vi "GFBuildMagTriggerWaveFormSLiC.vi"(1 "Li Trig Time":dbl, 2 "Li On Width":dbl, 4 "LED Trig Time":dbl, 6 "Invert":bool, 7 "LED On Width":dbl, 8 "error in":errorcluster, 9 "Enable Array":bool[](array[boolean])=[TRUE, TRUE, TRUE, TRUE, TRUE, TRUE, TRUE], 10 "Chan Delays":dbl[](array[numeric])=[-0.8, -0.9, -0.7] format="%.6f", 11 "task in":refnum<k21>="USB-MagAndTrigFire") -> (0 "error out":errorcluster, 3 "task out":refnum<k21>="USB-MagAndTrigFire", 5 "Digital Waveform Graph":digitalwaveform[](graph))   [LabVIEW 2016]
doc: "Magnet timing pulses should be input relative to fast fire pulse, at most 2 s behind (-2 to 0 s)"
uses:
  <vilib>/Waveform/DWDTOps.llb/DWDT Boolean Array to Digital.vi
  <resource>/objmgr/daqmx.rc
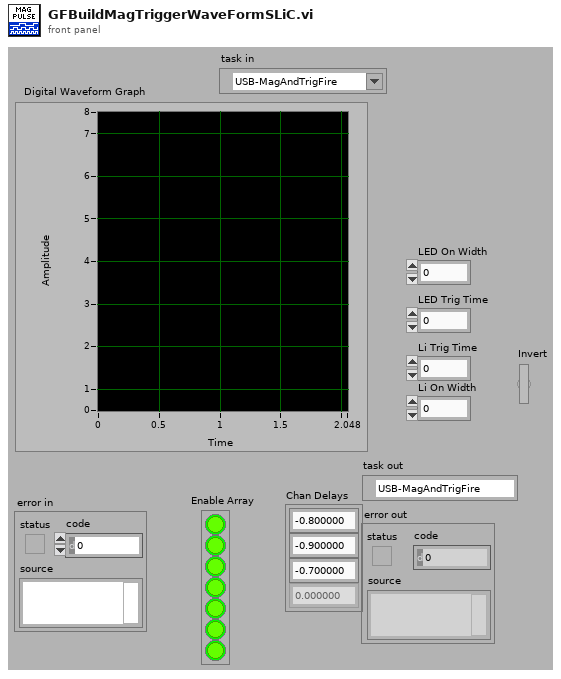
[diagram p1: front panel]
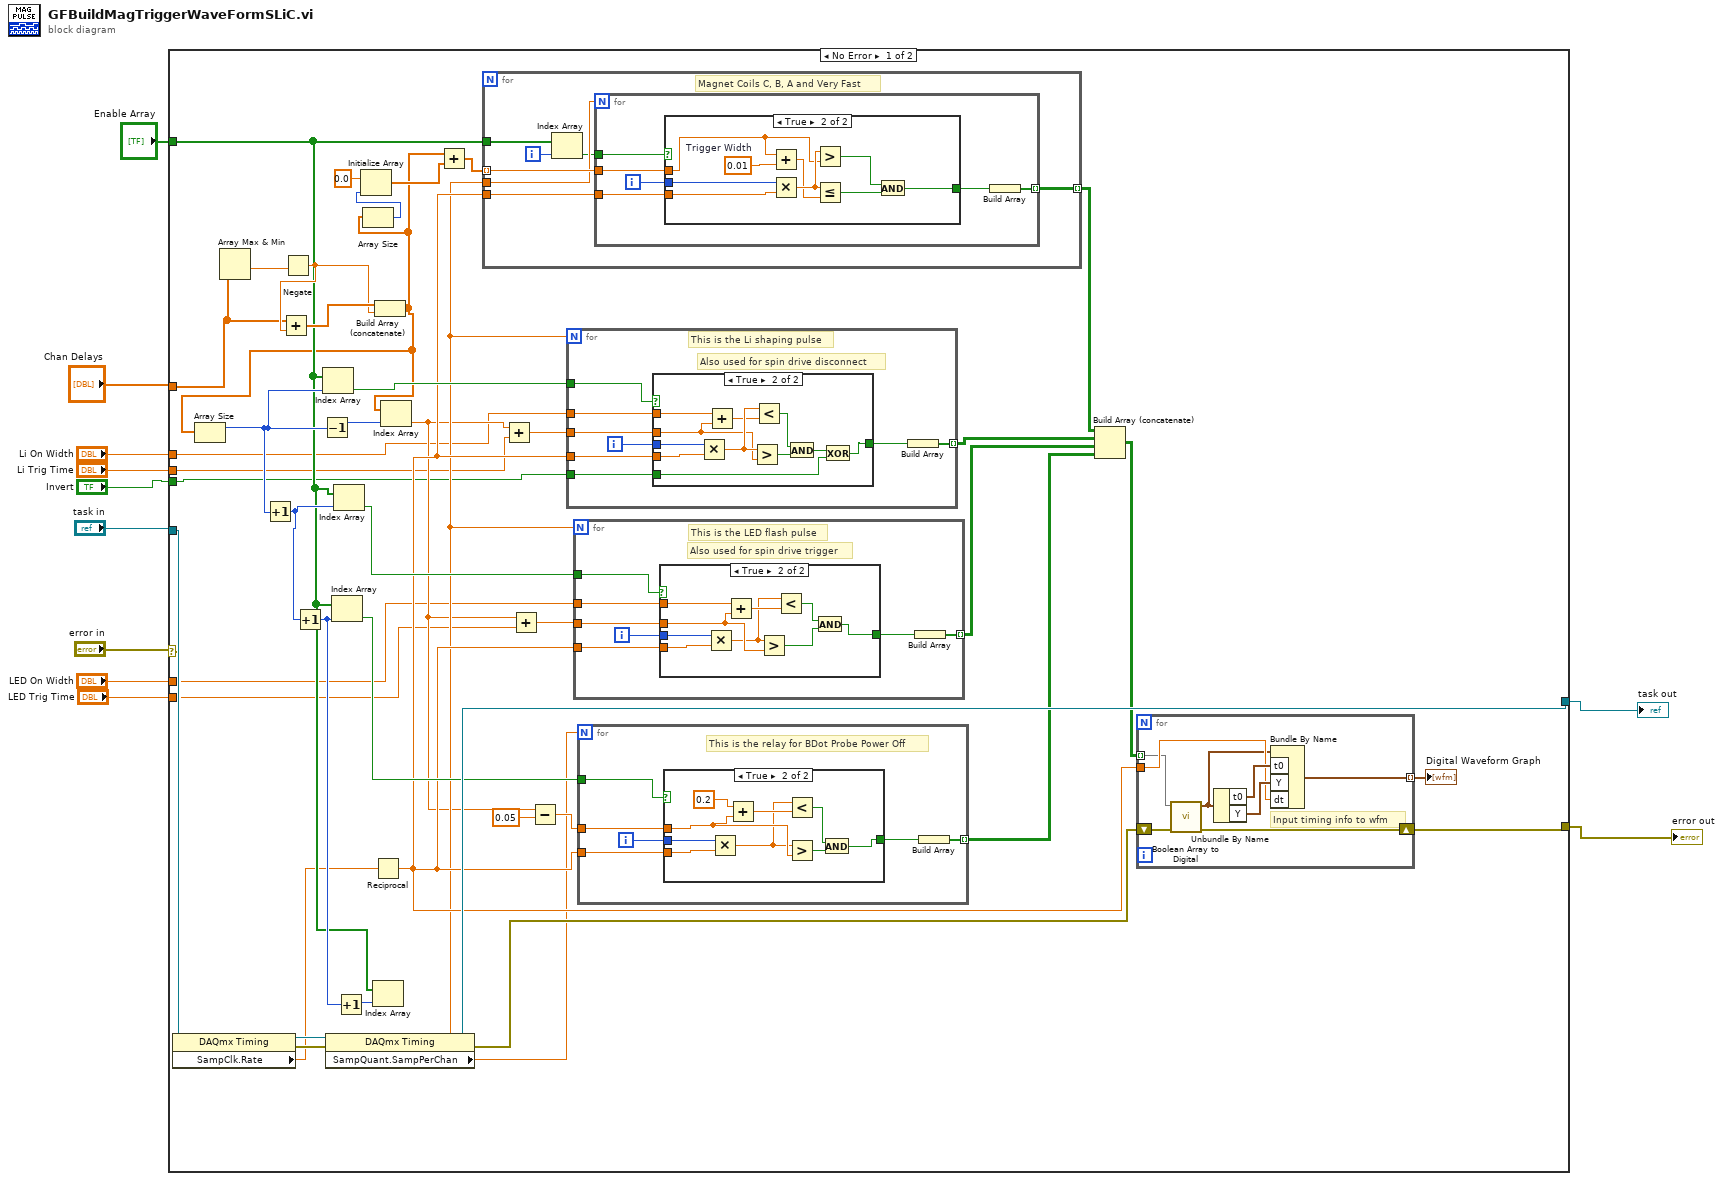
[diagram p0: block diagram]
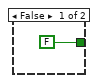
[diagram p2: hidden frame]
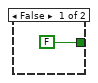
[diagram p3: hidden frame]
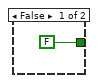
[diagram p4: hidden frame]
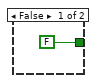
[diagram p5: hidden frame]
diagram:
  n1 = case shown="No Error" "error in" {
    selector: "error in" -> [w52 w140]
    tunnel: "task in" -> [w53 w141]
    tunnel: [w49 w141] -> w10
    tunnel: [w55 w140] -> w8
    tunnel: "Chan Delays" -> [w19 _]
    tunnel: "Enable Array" -> [w26 _]
    tunnel: "LED Trig Time" -> [w17 _]
    tunnel: "LED On Width" -> [w15 _]
    tunnel: "Li Trig Time" -> [w14 _]
    tunnel: "Li On Width" -> [w13 _]
    tunnel: "Invert" -> [w12 _]
    frame No Error {
      n2 = property class="DAQmx Timing"(reference=w53, error in=w52) -> (reference out=w51:refnum<k21>, error out=w50:errorcluster, "SampClk.Rate"=w25:dbl)
      n3 = Array Max & Min(array=w19) -> (min value=w45:dbl)  [unwired: 3 out]
      n4 = Negate(x=w45) -> (-x=w43:dbl)
      n5 = Add(x=w19, y=w43) -> (x+y=w44:dbl[])
      n6 = property class="DAQmx Timing"(reference=w51, error in=w50) -> (reference out=w49:refnum<k21>, error out=w37:errorcluster, "SampQuant.SampPerChan"=w29:dbl)
      n7 = Reciprocal(x=w25) -> (1/x=w33:dbl)
      n8 = Build Array (concatenate)(w44, w43) -> (w22:dbl[])
      n9 = Array Size(array=w22) -> (size(s)=w32:i32)
      n10 = Increment(x=w32) -> (x+1=w38:i32)
      n11 = Increment(x=w38) -> (x+1=w27:i32)
      n12 = Decrement(x=w32) -> (x-1=w48:i32)
      n13 = Index Array(array=w26, index=w32) -> (element=w42:bool)
      n14 = Index Array(array=w26, index=w27) -> (element=w36:bool)
      n15 = Index Array(array=w26, index=w38) -> (element=w40:bool)
      n16 = Increment(x=w27) -> (x+1=w28:i32)
      n17 = Array Size(array=w22) -> (size(s)=w21:i32)
      n18 = Initialize Array(0.0 ("element"), w21) -> (w23:dbl[])
      n19 = Index Array(array=w26, index=w28) -> ()  [unwired: 1 out]
      n20 = Index Array(array=w22, index=w48) -> (element=w18:dbl)
      n21 = Add(x=w22, y=w23) -> (x+y=w24:dbl[])
      n22 = for {
        tunnel: [w120] -> w47 mode=indexing
        tunnel: w24 -> [w123] mode=indexing
        tunnel: w33 -> [w122]
        tunnel: w29 -> [w121]
        tunnel: w26 -> [w119]
        i -> [w118]
        # "Magnet Coils C, B, A and Very Fast"
        n23 = Index Array(array=w119, index=w118) -> (element=w117:bool)
        n24 = for {
          N: w121 -> [_]
          tunnel: w123 -> [w128]
          tunnel: w122 -> [w129]
          tunnel: [w126] -> w120 mode=indexing
          tunnel: w117 -> [w124]
          i -> [w125]
          n25 = case shown="True" w124 {
            tunnel: w129 -> [_ w139]
            tunnel: w128 -> [_ w137]
            tunnel: [FALSE w132] -> w127
            tunnel: w125 -> [_ w131]
            frame False {
            }
            frame True {
              w136 = 0.01  # Trigger Width
              n26 = Add(x=w137, y=w136) -> (x+y=w135:dbl)
              n27 = Multiply(x=w131, y=w139) -> (x*y=w138:dbl)
              n28 = Greater?(x=w138, y=w137) -> (0:w134:bool)
              n29 = Less Or Equal?(x=w138, y=w135) -> (x <= y?=w133:bool)
              n30 = And(x=w134, y=w133) -> (x .and. y?=w132:bool)
            }
          }
          n31 = Build Array(w127) -> (w126:bool[])
        }
      }
      n32 = Add(x=w18, y=w14) -> (x+y=w35:dbl)
      n33 = Add(x=w18, y=w17) -> (x+y=w16:dbl)
      n34 = Subtract(x=w18, y=0.05) -> (x-y=w31:dbl)
      n35 = for {
        N: w29 -> [_]
        tunnel: w35 -> [w95]
        tunnel: w33 -> [w96]
        tunnel: [w94] -> w39 mode=indexing
        tunnel: w42 -> [w91]
        tunnel: w13 -> [w90]
        tunnel: w12 -> [w89]
        i -> [w93]
        # "Also used for spin drive disconnect"
        # "This is the Li shaping pulse"
        n36 = case shown="True" w91 {
          tunnel: w96 -> [_ w108]
          tunnel: w95 -> [_ w102]
          tunnel: w93 -> [_ w105]
          tunnel: [FALSE w99] -> w92
          tunnel: w90 -> [_ w101]
          tunnel: w89 -> [_ w98]
          frame False {
          }
          frame True {
            n37 = Multiply(x=w105, y=w108) -> (x*y=w104:dbl)
            n38 = Add(x=w101, y=w102) -> (x+y=w103:dbl)
            n39 = Greater?(x=w104, y=w102) -> (0:w107:bool)
            n40 = Less?(x=w104, y=w103) -> (x < y?=w106:bool)
            n41 = And(x=w106, y=w107) -> (x .and. y?=w100:bool)
            n42 = Exclusive Or(1:w98, 2:w100) -> (0:w99:bool)
          }
        }
        n43 = Build Array(w92) -> (w94:bool[])
      }
      n44 = for {
        N: w29 -> [_]
        tunnel: w16 -> [w77]
        tunnel: w33 -> [w78]
        tunnel: [w76] -> w41 mode=indexing
        tunnel: w40 -> [w73]
        tunnel: w15 -> [w72]
        i -> [w75]
        # "Also used for spin drive trigger"
        # "This is the LED flash pulse"
        n45 = case shown="True" w73 {
          tunnel: w78 -> [_ w88]
          tunnel: w77 -> [_ w82]
          tunnel: w75 -> [_ w87]
          tunnel: [FALSE w85] -> w74
          tunnel: w72 -> [_ w80]
          frame False {
          }
          frame True {
            n46 = Multiply(x=w87, y=w88) -> (x*y=w81:dbl)
            n47 = Add(x=w80, y=w82) -> (x+y=w86:dbl)
            n48 = Greater?(x=w81, y=w82) -> (0:w83:bool)
            n49 = Less?(x=w81, y=w86) -> (x < y?=w84:bool)
            n50 = And(x=w84, y=w83) -> (x .and. y?=w85:bool)
          }
        }
        n51 = Build Array(w74) -> (w76:bool[])
      }
      n52 = for {
        N: w29 -> [_]
        tunnel: w31 -> [w60]
        tunnel: w33 -> [w61]
        tunnel: [w59] -> w34 mode=indexing
        tunnel: w36 -> [w56]
        i -> [w58]
        # "This is the relay for BDot Probe Power Off"
        n53 = case shown="True" w56 {
          tunnel: w61 -> [_ w71]
          tunnel: w60 -> [_ w65]
          tunnel: w58 -> [_ w67]
          tunnel: [FALSE w69] -> w57
          frame False {
          }
          frame True {
            n54 = Multiply(x=w67, y=w71) -> (x*y=w63:dbl)
            n55 = Add(x=0.2, y=w65) -> (x+y=w64:dbl)
            n56 = Less?(x=w63, y=w64) -> (x < y?=w68:bool)
            n57 = Greater?(x=w63, y=w65) -> (0:w70:bool)
            n58 = And(x=w68, y=w70) -> (x .and. y?=w69:bool)
          }
        }
        n59 = Build Array(w57) -> (w59:bool[])
      }
      n60 = Build Array (concatenate)(w47, w39, w41, w34) -> (w46:bool[][][])
      n61 = for {
        shift-right: [w116] -> w55
        shift-left: w37 -> [w115]
        tunnel: w46 -> [w109] mode=indexing
        tunnel: [w110] -> w54 mode=indexing
        tunnel: w33 -> [w112]
        # "Input timing info to wfm"
        n62 = call-poly <vilib>:"Boolean Array to Digital.vi"("error in (no error)"=w115, "boolean array"=w109) -> ("error out"=w116:errorcluster, "digital waveform"=w111:digitalwaveform)  [unwired: 8 in]
        n63 = Unbundle By Name(w111) -> ("t0"=w114:timestamp, "Y"=w113:digitaldata)
        n64 = Bundle By Name(cluster=w111, "t0"=w114, "Y"=w113, "dt"=w112) -> (w110:digitalwaveform)
      }
      "Digital Waveform Graph" <- w54
    }
    frame Error {
    }
  }
  "error out" <- w8
  "task out" <- w10
